vi "易损件管理.vi"() -> ()   [LabVIEW 2017]
uses:
  <vilib>/addons/database/Connection.llb/DB Tools Open Connec (String).vi
  <vilib>/addons/database/Connection.llb/Conn Execute.vi
  <vilib>/addons/database/Recordset.llb/Rec Fetch Recordset Data (R).vi
  <vilib>/addons/database/Recordset.llb/Rec Destroy - Connection.vi
  <vilib>/addons/database/NI_Database_API.lvlib
panel:
  out "易损件":string[][](table)
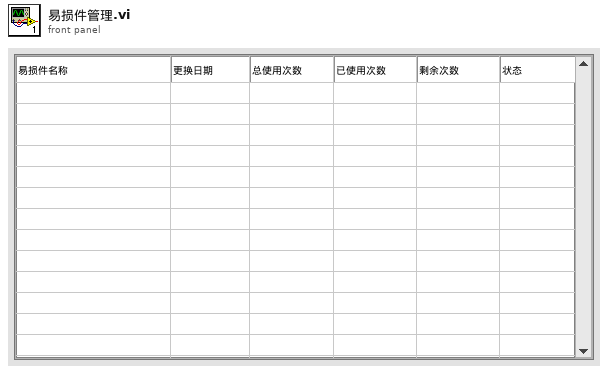
[diagram p1: front panel]
types:
  T1 = typedef "NI_Database_API.lvlib/Conn ObjectReference.ctl" = refnum<k1>
  T2 = typedef "NI_Database_API.lvlib/Rec ObjectReference.ctl" = refnum<k1>
  T3 = typedef "LVPoint32TypeDef.ctl" = cluster{"Horizontal":i32, "Vertical":i32}
  T4 = typedef "LVRowAndColumnTypeDef.ctl" = cluster{"Row":i32, "Column":i32}
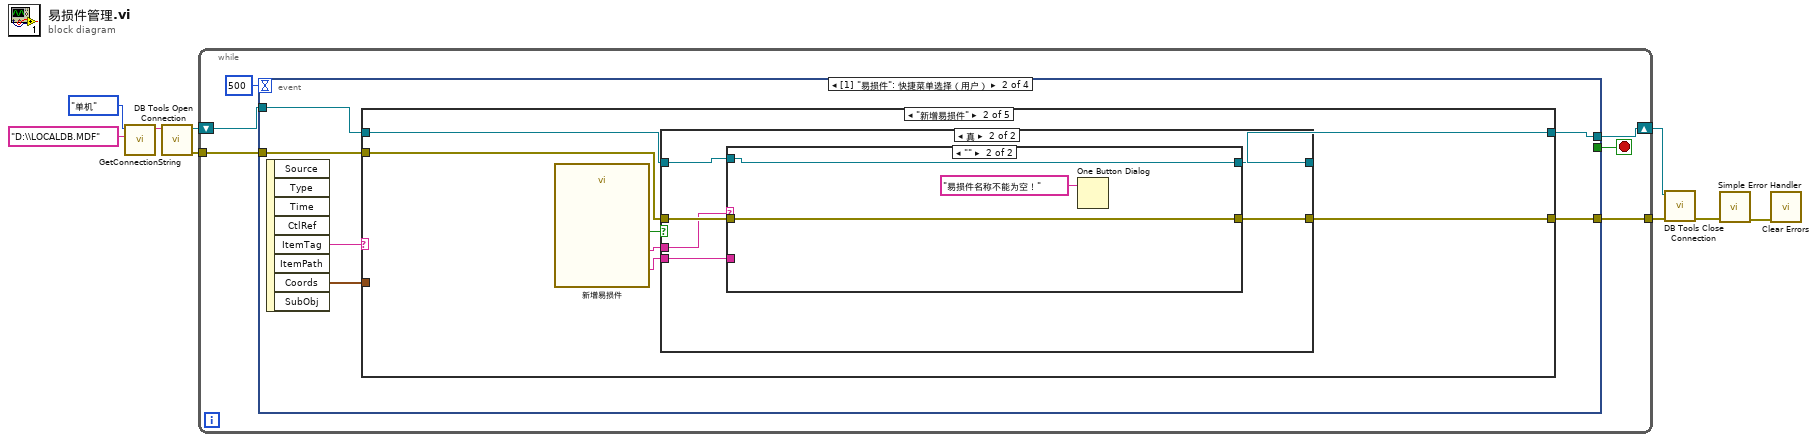
[diagram p0: block diagram]
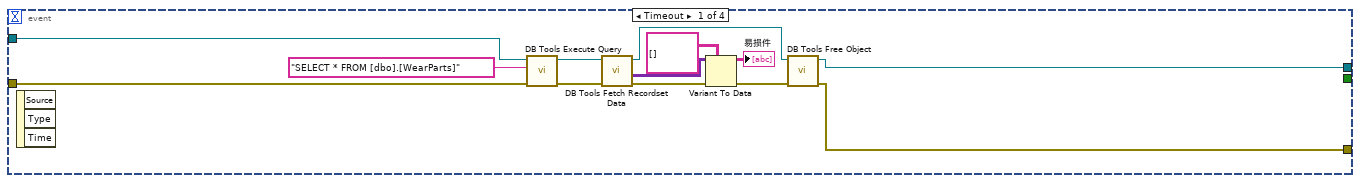
[diagram p2: hidden frame]
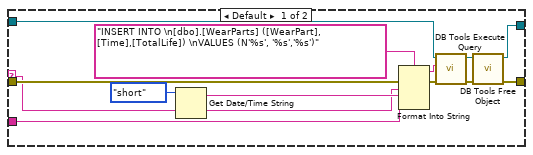
[diagram p5: hidden frame]
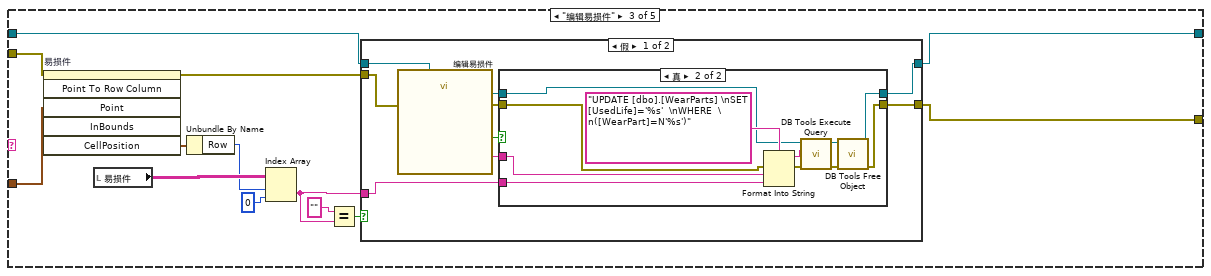
[diagram p6: hidden frame]
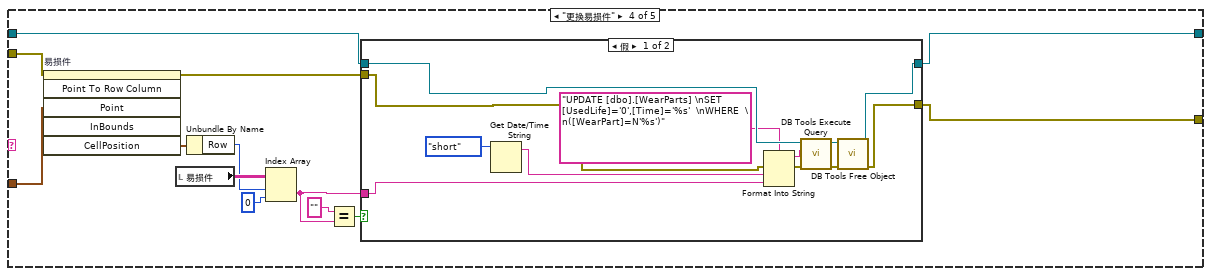
[diagram p9: hidden frame]
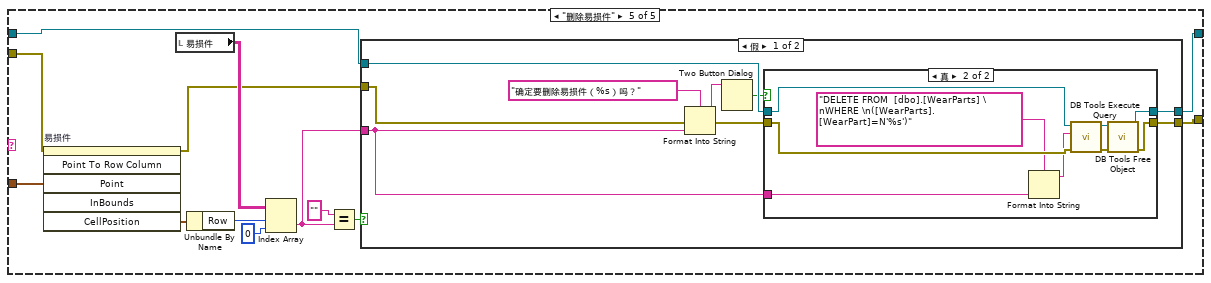
[diagram p11: hidden frame]
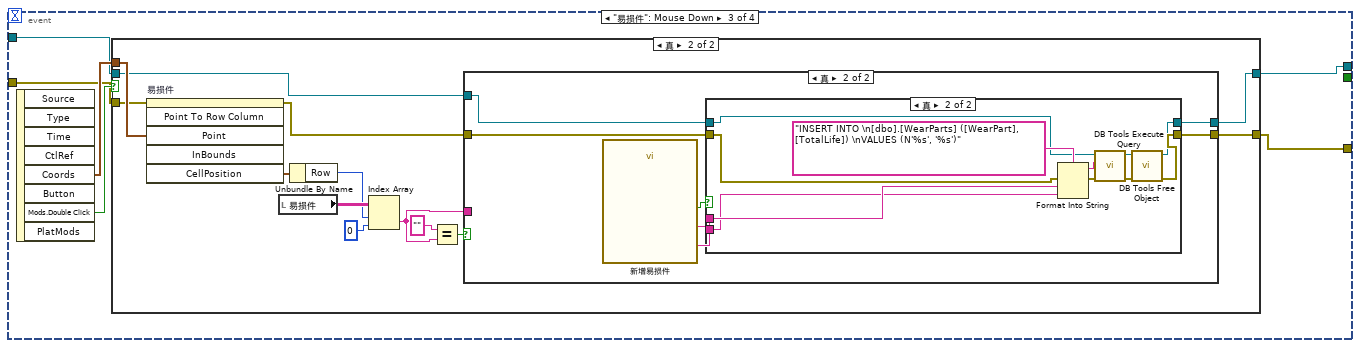
[diagram p14: hidden frame]
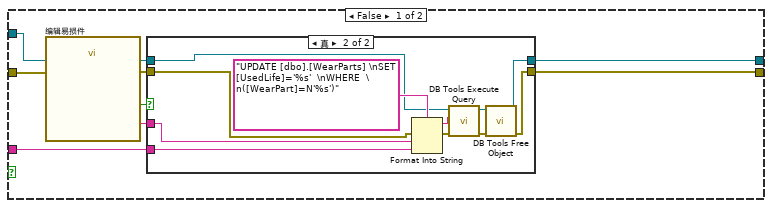
[diagram p16: hidden frame]
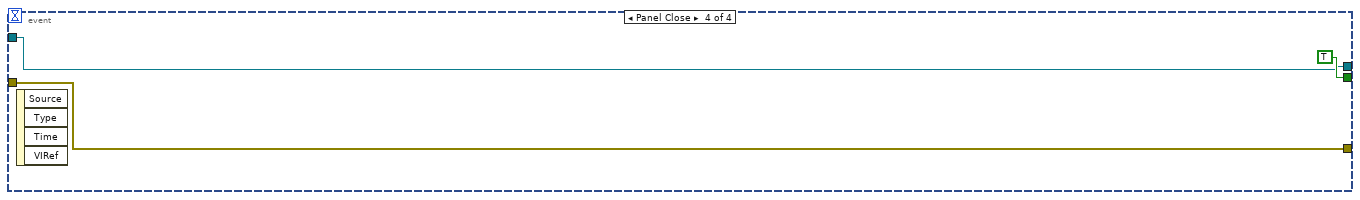
[diagram p19: hidden frame]
diagram:
  n1 = call "GetConnectionString.vi"("Database Name"="D:\\LOCALDB.MDF", "连接模式"=enum16{"单机", "联网"}."单机") -> ("连接字符串"=w7:string)  [unwired: 4 in, 1 out]
  n2 = call-poly <vilib>:"DB Tools Open Connection.vi"("connection information"=w7) -> ("error out"=w3:errorcluster, "connection reference"=w4:T1)  [unwired: 7 in]
  n3 = while {
    tunnel: [w14] -> w9
    tunnel: w3 -> [w11]
    shift-right: [w13] -> w8
    shift-left: w4 -> [w12]
    stop <- w15 stop-if-true
    n4 = event shown="[1] \"易损件\": 快捷菜单选择（用户）" {
      selector: _ -> [_ _ _ _]
      dyn-events: _ -> [_ _ _ _]
      timeout: 500 -> [_ _ _ _]
      tunnel: [_ _ _ TRUE] -> w15
      tunnel: [w16 w33 w166 w228] -> w14
      tunnel: [w17 w32 w167 w229] -> w13
      tunnel: w12 -> [w22 w31 w168 w229]
      tunnel: w11 -> [w21 w30 w169 w228]
      event Timeout {
        n5 = event-data() -> ()  [unwired: 1 in, 3 out]
        n6 = call-poly <vilib>:"DB Tools Execute Query.vi"("error in (no error)"=w21, "SQL query"="SELECT * FROM [dbo].[WearParts]", "connection reference"=w22) -> ("error out"=w27:errorcluster, "recordset reference"=w26:T2)  [unwired: 5 in]
        n7 = call-poly <vilib>:"DB Tools Fetch Recordset Data.vi"("error in (no error)"=w27, "recordset reference"=w26) -> ("error out"=w25:errorcluster, "recordset data"=w24:variant[][], "recordset reference out"=w19:T2)  [unwired: 3 in]
        n8 = Variant To Data(error in=w25, type=string[][] [], Variant=w24) -> (data=→"易损件":string[][], error out=w18:errorcluster)
        n9 = call-poly <vilib>:"DB Tools Free Object.vi"("error in (no error)"=w18, "recordset reference"=w19) -> ("error out"=w16:errorcluster, "connection reference"=w17:T1)  [unwired: 8 in]
      }
      event "易损件": Shortcut Menu Selection (User) {
        n10 = event-data() -> ("ItemTag"=w34:string, "Coords"=w29:T3)  [unwired: 1 in, 6 out]
        n11 = case shown="\"新增易损件\"" w34 {
          tunnel: [w35 w40 w68 w104 w132] -> w33
          tunnel: [w36 w39 w69 w105 w133] -> w32
          tunnel: w31 -> [w36 w38 w73 w109 w134]
          tunnel: w30 -> [w35 w37 w72 w108 w131]
          tunnel: w29 -> [_ _ w80 w116 w138]
          frame "假", Default {
          }
          frame "新增易损件" {
            n12 = call "新增易损件"() -> ("易损件总使用次数"=w42:string, "易损件名称"=w43:string, "确定"=w41:bool)  [unwired: 16 in, 1 out]
            n13 = case shown="真" w41 {
              tunnel: w43 -> [_ w46]
              tunnel: w42 -> [_ w47]
              tunnel: [w44 w51] -> w40
              tunnel: [w45 w50] -> w39
              tunnel: w38 -> [w45 w49]
              tunnel: w37 -> [w44 w48]
              frame False {
              }
              frame True {
                n14 = case shown="\"\"" w46 {
                  selector: w46 -> [w52 _]
                  tunnel: [w59 w66] -> w51
                  tunnel: [w58 w67] -> w50
                  tunnel: w49 -> [w57 w67]
                  tunnel: w48 -> [w56 w66]
                  tunnel: w47 -> [w55 _]
                  frame Default {
                    n15 = Get Date/Time String(date format (0)=enum16{"short", "long", "abbreviated"}."short" ("日期格式(0)")) -> (date string=w53:string)  [unwired: 2 in, 1 out]
                    n16 = Format Into String(format string="INSERT INTO \n[dbo].[WearParts] ([WearPart], [Time],[TotalLife]) \nVALUES (N'%s', '%s','%s')" ("格式字符串"), error in=w56, w52, w53, w55) -> (resulting string=w63:string, error out=w60:errorcluster)  [unwired: 1 in]
                    n17 = call-poly <vilib>:"DB Tools Execute Query.vi"("error in (no error)"=w60, "SQL query"=w63, "connection reference"=w57) -> ("error out"=w62:errorcluster, "recordset reference"=w61:T2)  [unwired: 5 in]
                    n18 = call-poly <vilib>:"DB Tools Free Object.vi"("error in (no error)"=w62, "recordset reference"=w61) -> ("error out"=w59:errorcluster, "connection reference"=w58:T1)  [unwired: 8 in]
                  }
                  frame "" {
                    n19 = One Button Dialog(message="易损件名称不能为空！" ("消息")) -> ()  [unwired: 1 in, 1 out]
                  }
                }
              }
            }
          }
          frame "编辑易损件" {
            n20 = invoke on="易损件" class="Tbl (严格)" method="Point To Row Column"(error in=w72, "Point"=w80) -> (error out=w71:errorcluster, "CellPosition"=w77:T4)  [unwired: 4 in, 4 out]
            n21 = local read "易损件"() -> (w76:string[][])
            n22 = Unbundle By Name(w77) -> ("Row"=w75:i32)
            n23 = Index Array(array=w76, index (row)=w75, index (col)=0 ("禁用的索引 (列)")) -> (element=w70:string)
            n24 = Equal?(x="" ("元素"), y=w70) -> (x = y?=w74:bool)
            n25 = case shown="假" w74 {
              tunnel: w73 -> [w87 w103]
              tunnel: w71 -> [w86 w102]
              tunnel: w70 -> [w83 _]
              tunnel: [w82 w103] -> w69
              tunnel: [w81 w102] -> w68
              frame False {
                n26 = call "编辑易损件"("error in (no error)"=w86) -> ("使用次数"=w84:string, "确定"=w88:bool, "error out"=w85:errorcluster)  [unwired: 16 in]
                n27 = case shown="真" w88 {
                  tunnel: w87 -> [w90 w96]
                  tunnel: w85 -> [w89 w95]
                  tunnel: w84 -> [_ w94]
                  tunnel: w83 -> [_ w93]
                  tunnel: [w90 w92] -> w82
                  tunnel: [w89 w91] -> w81
                  frame False {
                  }
                  frame True {
                    n28 = Format Into String(format string="UPDATE [dbo].[WearParts] \nSET [UsedLife]='%s'  \nWHERE  \n([WearPart]=N'%s')" ("格式字符串"), error in=w95, w94, w93) -> (resulting string=w100:string, error out=w97:errorcluster)  [unwired: 1 in]
                    n29 = call-poly <vilib>:"DB Tools Execute Query.vi"("error in (no error)"=w97, "SQL query"=w100, "connection reference"=w96) -> ("error out"=w99:errorcluster, "recordset reference"=w98:T2)  [unwired: 5 in]
                    n30 = call-poly <vilib>:"DB Tools Free Object.vi"("error in (no error)"=w99, "recordset reference"=w98) -> ("error out"=w91:errorcluster, "connection reference"=w92:T1)  [unwired: 8 in]
                  }
                }
              }
              frame True {
              }
            }
          }
          frame "更换易损件" {
            n31 = invoke on="易损件" class="Tbl (严格)" method="Point To Row Column"(error in=w108, "Point"=w116) -> (error out=w107:errorcluster, "CellPosition"=w113:T4)  [unwired: 4 in, 4 out]
            n32 = local read "易损件"() -> (w112:string[][])
            n33 = Unbundle By Name(w113) -> ("Row"=w111:i32)
            n34 = Index Array(array=w112, index (row)=w111, index (col)=0 ("禁用的索引 (列)")) -> (element=w106:string)
            n35 = Equal?(x="" ("元素"), y=w106) -> (x = y?=w110:bool)
            n36 = case shown="假" w110 {
              tunnel: w109 -> [w128 w130]
              tunnel: w107 -> [w124 w129]
              tunnel: w106 -> [w127 _]
              tunnel: [w126 w130] -> w105
              tunnel: [w125 w129] -> w104
              frame False {
                n37 = Get Date/Time String(date format (0)=enum16{"short", "long", "abbreviated"}."short" ("日期格式(0)")) -> (date string=w118:string)  [unwired: 2 in, 1 out]
                n38 = Format Into String(format string="UPDATE [dbo].[WearParts] \nSET [UsedLife]='0',[Time]='%s'  \nWHERE  \n([WearPart]=N'%s')" ("格式字符串"), error in=w124, w118, w127) -> (resulting string=w122:string, error out=w119:errorcluster)  [unwired: 1 in]
                n39 = call-poly <vilib>:"DB Tools Execute Query.vi"("error in (no error)"=w119, "SQL query"=w122, "connection reference"=w128) -> ("error out"=w121:errorcluster, "recordset reference"=w120:T2)  [unwired: 5 in]
                n40 = call-poly <vilib>:"DB Tools Free Object.vi"("error in (no error)"=w121, "recordset reference"=w120) -> ("error out"=w125:errorcluster, "connection reference"=w126:T1)  [unwired: 8 in]
              }
              frame True {
              }
            }
          }
          frame "删除易损件" {
            n41 = invoke on="易损件" class="Tbl (严格)" method="Point To Row Column"(error in=w131, "Point"=w138) -> (error out=w135:errorcluster, "CellPosition"=w141:T4)  [unwired: 4 in, 4 out]
            n42 = local read "易损件"() -> (w140:string[][])
            n43 = Unbundle By Name(w141) -> ("Row"=w139:i32)
            n44 = Index Array(array=w140, index (row)=w139, index (col)=0 ("禁用的索引 (列)")) -> (element=w136:string)
            n45 = Equal?(x="" ("元素"), y=w136) -> (x = y?=w137:bool)
            n46 = case shown="假" w137 {
              tunnel: w136 -> [w144 _]
              tunnel: w135 -> [w151 w164]
              tunnel: w134 -> [w149 w165]
              tunnel: [w147 w165] -> w133
              tunnel: [w146 w164] -> w132
              frame False {
                n47 = Format Into String(format string="确定要删除易损件（%s）吗？" ("格式字符串"), error in=w151, w144) -> (resulting string=w150:string, error out=w148:errorcluster)  [unwired: 1 in]
                n48 = Two Button Dialog(message=w150) -> (T button?=w145:bool)  [unwired: 2 in]
                n49 = case shown="真" w145 {
                  tunnel: w149 -> [w154 w163]
                  tunnel: w148 -> [w153 w162]
                  tunnel: [w154 w159] -> w147
                  tunnel: [w153 w158] -> w146
                  tunnel: w144 -> [_ w156]
                  frame False {
                  }
                  frame True {
                    n50 = Format Into String(format string="DELETE FROM  [dbo].[WearParts] \nWHERE \n([WearParts].[WearPart]=N'%s')" ("格式字符串"), w156) -> (resulting string=w155:string)  [unwired: 2 in, 1 out]
                    n51 = call-poly <vilib>:"DB Tools Execute Query.vi"("error in (no error)"=w162, "SQL query"=w155, "connection reference"=w163) -> ("error out"=w161:errorcluster, "recordset reference"=w160:T2)  [unwired: 5 in]
                    n52 = call-poly <vilib>:"DB Tools Free Object.vi"("error in (no error)"=w161, "recordset reference"=w160) -> ("error out"=w158:errorcluster, "connection reference"=w159:T1)  [unwired: 8 in]
                  }
                }
              }
              frame True {
              }
            }
          }
        }
      }
      event "易损件": Mouse Down {
        n53 = event-data() -> ("Coords"=w170:T3, "Mods.Double Click"=w171:bool)  [unwired: 1 in, 6 out]
        n54 = case shown="真" w171 {
          tunnel: w170 -> [_ w181]
          tunnel: w169 -> [w172 w180]
          tunnel: w168 -> [w173 w177]
          tunnel: [w173 w176] -> w167
          tunnel: [w172 w175] -> w166
          frame False {
          }
          frame True {
            n55 = invoke on="易损件" class="Tbl (严格)" method="Point To Row Column"(error in=w180, "Point"=w181) -> (error out=w178:errorcluster, "CellPosition"=w184:T4)  [unwired: 4 in, 4 out]
            n56 = local read "易损件"() -> (w183:string[][])
            n57 = Unbundle By Name(w184) -> ("Row"=w182:i32)
            n58 = Index Array(array=w183, index (row)=w182, index (col)=0 ("禁用的索引 (列)")) -> (element=w174:string)
            n59 = Equal?(x="" ("元素"), y=w174) -> (x = y?=w179:bool)
            n60 = case shown="真" w179 {
              tunnel: w178 -> [w193 w211]
              tunnel: w177 -> [w194 w210]
              tunnel: [w192 w209] -> w176
              tunnel: [w191 w208] -> w175
              tunnel: w174 -> [w190 _]
              frame False {
                n61 = call "编辑易损件"("error in (no error)"=w193) -> ("使用次数"=w187:string, "确定"=w189:bool, "error out"=w188:errorcluster)  [unwired: 16 in]
                n62 = case shown="真" w189 {
                  tunnel: w194 -> [w196 w202]
                  tunnel: w188 -> [w195 w201]
                  tunnel: w187 -> [_ w200]
                  tunnel: w190 -> [_ w199]
                  tunnel: [w196 w198] -> w192
                  tunnel: [w195 w197] -> w191
                  frame False {
                  }
                  frame True {
                    n63 = Format Into String(format string="UPDATE [dbo].[WearParts] \nSET [UsedLife]='%s'  \nWHERE  \n([WearPart]=N'%s')" ("格式字符串"), error in=w201, w200, w199) -> (resulting string=w206:string, error out=w203:errorcluster)  [unwired: 1 in]
                    n64 = call-poly <vilib>:"DB Tools Execute Query.vi"("error in (no error)"=w203, "SQL query"=w206, "connection reference"=w202) -> ("error out"=w205:errorcluster, "recordset reference"=w204:T2)  [unwired: 5 in]
                    n65 = call-poly <vilib>:"DB Tools Free Object.vi"("error in (no error)"=w205, "recordset reference"=w204) -> ("error out"=w197:errorcluster, "connection reference"=w198:T1)  [unwired: 8 in]
                  }
                }
              }
              frame True {
                n66 = call "新增易损件"() -> ("易损件总使用次数"=w213:string, "易损件名称"=w214:string, "确定"=w212:bool)  [unwired: 16 in, 1 out]
                n67 = case shown="真" w212 {
                  tunnel: w214 -> [_ w226]
                  tunnel: w213 -> [_ w225]
                  tunnel: [w215 w220] -> w208
                  tunnel: [w216 w219] -> w209
                  tunnel: w210 -> [w216 w218]
                  tunnel: w211 -> [w215 w217]
                  frame False {
                  }
                  frame True {
                    n68 = Format Into String(format string="INSERT INTO \n[dbo].[WearParts] ([WearPart], [TotalLife]) \nVALUES (N'%s', '%s')" ("格式字符串"), error in=w217, w226, w225) -> (resulting string=w224:string, error out=w221:errorcluster)  [unwired: 1 in]
                    n69 = call-poly <vilib>:"DB Tools Execute Query.vi"("error in (no error)"=w221, "SQL query"=w224, "connection reference"=w218) -> ("error out"=w223:errorcluster, "recordset reference"=w222:T2)  [unwired: 5 in]
                    n70 = call-poly <vilib>:"DB Tools Free Object.vi"("error in (no error)"=w223, "recordset reference"=w222) -> ("error out"=w220:errorcluster, "connection reference"=w219:T1)  [unwired: 8 in]
                  }
                }
              }
            }
          }
        }
      }
      event Panel Close {
        n71 = event-data() -> ()  [unwired: 1 in, 4 out]
      }
    }
  }
  n72 = call <vilib>:"DB Tools Close Connection.vi"("error in (no error)"=w9, "connection reference"=w8) -> ("error out"=w1:errorcluster)  [unwired: 5 in]
  n73 = call <vilib>:"Simple Error Handler.vi"("error in (no error)"=w1) -> ("error out"=w2:errorcluster)  [unwired: 4 in, 4 out]
  n74 = call <vilib>:"Clear Errors.vi"("error in (no error)"=w2) -> ()  [unwired: 5 in, 2 out]
